vi "Write Ign Data.vi"(8 "error in (no error)":errorcluster, 9 "NodeIDs":string[](array[string]), 10 "Control Ref":refnum<vi>, 11 "OPC UA client refnum":T1) -> (0 "error out":errorcluster, 3 "OPC UA client refnum":T1)   [LabVIEW 2019, in "Ignition.lvlib"]
uses:
  Ignition.lvlib
  <vilib>/OPCUA/controls/OPC UA Client Refnum.ctl
  <vilib>/OPCUA/controls/Write Status.ctl
  <vilib>/OPCUA/controls/Write Variant Request.ctl
  <vilib>/OPCUA/controls/NodeId.ctl
  <vilib>/OPCUA/client/Multiple Write Variant.vi
  <vilib>/OPCUA/NI OPC UA Client.lvlib
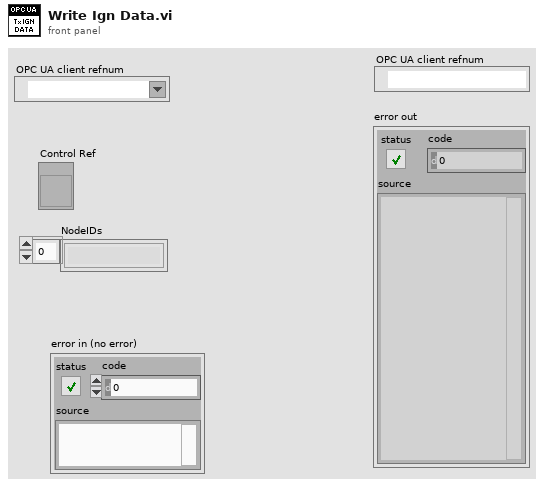
[diagram p1: front panel]
types:
  T1 = typedef "OPC UA Client Refnum.ctl" = refnum<k21>
  T2 = typedef "Write Status.ctl" = u32
  T3 = typedef "Write Variant Request.ctl" = cluster{"node ID":T4, "value":variant, "timestamp (current time)":timestamp, "node status":T2}
  T4 = typedef "NodeId.ctl" = string
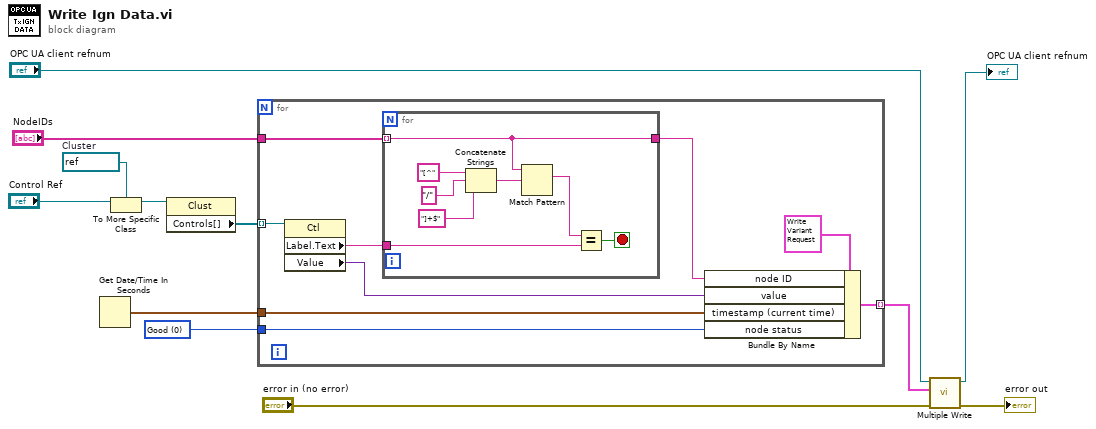
[diagram p0: block diagram]
diagram:
  w10 = refnum<vi> refnum  # Cluster
  w11 = T2 0 items=["Good"=0, "Uncertain"=1073741824, "Uncertain_InitialValue"=1083310080, "Uncertain_LastUsableValue"=1083179008, "Uncertain_SensorNotAccurate"=1083375616, "Uncertain_EngineeringUnitsExceeded"=1083441152, "Bad"=2147483648, "Bad_NoCommunication"=2150694912, "Bad_NotReadable"=2151284736, "Bad_NotWritable"=2151350272, "Bad_OutOfRange"=2151415808, "Bad_WaitingForInitialData"=2150760448] ("node status")
  n1 = Get Date/Time In Seconds() -> (seconds since 1Jan1904=w12:timestamp)
  n2 = To More Specific Class(target class=w10, reference="Control Ref") -> (specific class reference=w9:refnum<vi>)  [unwired: 1 in, 1 out]
  n3 = property class="Clust"(reference=w9) -> ("Controls[]"=w8:refnum<vi>[])  [unwired: 1 in, 2 out]
  n4 = for {
    tunnel: w8 -> [w21] mode=indexing
    tunnel: [w18] -> w7 mode=indexing
    tunnel: w12 -> [w17]
    tunnel: w11 -> [w15]
    tunnel: "NodeIDs" -> [w13]
    n5 = property class="Ctl"(reference=w21) -> ("Label.Text"=w20:string, "Value"=w14:variant)  [unwired: 1 in, 2 out]
    n6 = for {
      tunnel: w20 -> [w29]
      tunnel: w13 -> [w24] mode=indexing
      tunnel: [w24] -> w16
      stop <- w28 stop-if-true
      n7 = Concatenate Strings("[^" ("string"), "/" ("Deliminated Char"), "]+$" ("string")) -> (w27:string)
      n8 = Match Pattern(string=w24, regular expression=w27) -> (match substring=w23:string)  [unwired: 1 in, 3 out]
      n9 = Equal?(x=w23, y=w29) -> (x = y?=w28:bool)
    }
    n10 = Bundle By Name(cluster=T3 {"node ID"="", "value"=variant, "timestamp (current time)"=timestamp(0 s since 1904-01-01), "node status"=0} ("request"), "node ID"=w16, "value"=w14, "timestamp (current time)"=w17, "node status"=w15) -> (w18:T3)
  }
  n11 = call-poly <vilib>:"Multiple Write.vi"("error in (no error)"="error in (no error)", "requests"=w7, "OPC UA client refnum in"="OPC UA client refnum") -> ("error out"=→"error out":errorcluster, "OPC UA client refnum out"=→"OPC UA client refnum":T1)  [unwired: 5 in, 2 out]
